vi "获取测试项目和点数.vi"(10 "Item&Count1":string[][](array[string])=[["DCR", "1"], ["DCV", "2"], ["ACV1", "4"], ["ACV2", "4"], ["DCI", "6"], ["ACI", "3"]], 11 "Item":refnum<vi>[](array[refnum])) -> (1 "测量项目":string[](array[string]), 3 "测量点数":i32[](array[numeric]))   [LabVIEW 2020]
panel:
  out "Item&Count2":string[][](array[string])
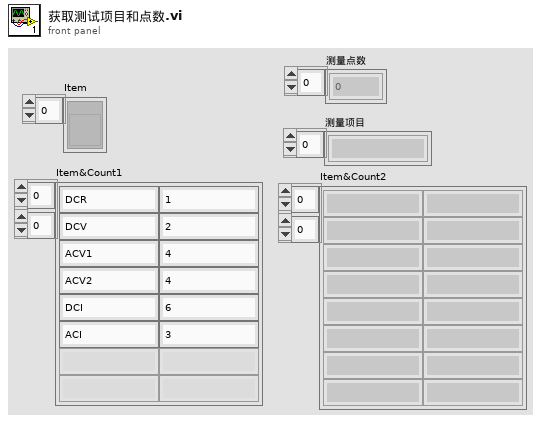
[diagram p1: front panel]
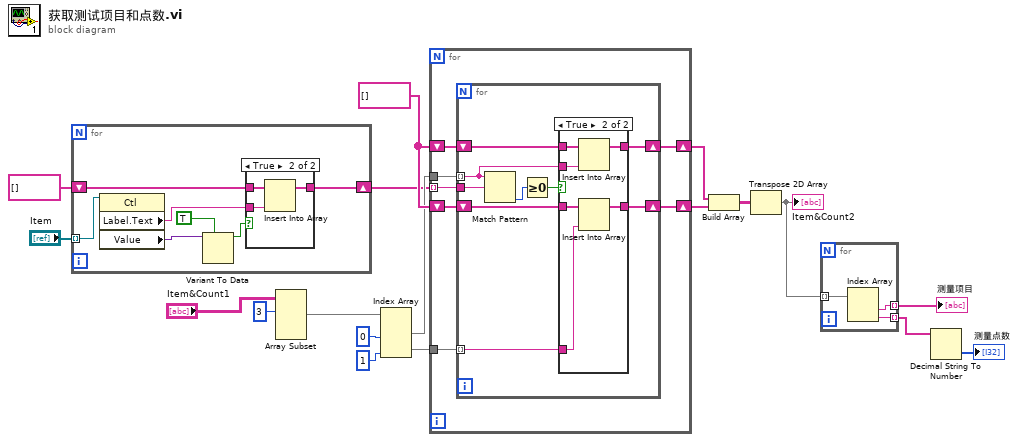
[diagram p0: block diagram]
diagram:
  w15 = string[] [] ("数组")
  n1 = for {
    shift-right: [w20] -> w11
    shift-left: string[] [] ("数组") -> [w21]
    tunnel: "Item" -> [w19] mode=indexing
    n2 = property class="Ctl"(reference=w19) -> ("Label.Text"=w22:string, "Value"=w25:variant)  [unwired: 1 in, 2 out]
    n3 = Variant To Data(type=TRUE, Variant=w25) -> (data=w23:bool)  [unwired: 1 in, 1 out]
    n4 = case shown="True" w23 {
      tunnel: w22 -> [_ w28]
      tunnel: w21 -> [w26 w29]
      tunnel: [w26 w27] -> w20
      frame False {
      }
      frame True {
        n5 = Insert Into Array(array=w29, new element=w28) -> (w27:string[])  [unwired: 1 in]
      }
    }
  }
  n6 = Array Subset(array="Item&Count1", index (row)=3 ("索引")) -> (w5:string[][])  [unwired: 3 in]
  n7 = Index Array(array=w5, index (col) #1=0 ("禁用的索引 (列)"), index (col) #2=1 ("索引 (列)")) -> (element #1=w12:string[], element #2=w14:string[])  [unwired: 2 in]
  n8 = for {
    tunnel: w11 -> [w36] mode=indexing
    tunnel: w12 -> [w35]
    shift-right: [w34] -> w16
    shift-left: w15 -> [w33]
    shift-right: [w31] -> w17
    shift-left: w15 -> [w32]
    tunnel: w14 -> [w30]
    n9 = for {
      tunnel: w36 -> [w45]
      tunnel: w35 -> [w41] mode=indexing
      shift-right: [w40] -> w34
      shift-left: w33 -> [w42]
      shift-right: [w38] -> w31
      shift-left: w32 -> [w39]
      tunnel: w30 -> [w37] mode=indexing
      n10 = Match Pattern(string=w41, regular expression=w45) -> (offset past match=w44:i32)  [unwired: 1 in, 3 out]
      n11 = Greater Or Equal To 0?(x=w44) -> (x >= 0?=w43:bool)
      n12 = case shown="True" w43 {
        tunnel: w42 -> [w47 w53]
        tunnel: w41 -> [_ w52]
        tunnel: [w47 w51] -> w40
        tunnel: w39 -> [w46 w50]
        tunnel: [w46 w49] -> w38
        tunnel: w37 -> [_ w48]
        frame False {
        }
        frame True {
          n13 = Insert Into Array(array=w53, new element=w52) -> (w51:string[])  [unwired: 1 in]
          n14 = Insert Into Array(array=w50, new element=w48) -> (w49:string[])  [unwired: 1 in]
        }
      }
    }
  }
  n15 = Build Array(w16, w17) -> (w18:string[][])
  n16 = Transpose 2D Array(2D array=w18) -> (transposed array=w4:string[][])
  "Item&Count2" <- w4
  n17 = for {
    tunnel: w4 -> [w56] mode=indexing
    tunnel: [w55] -> w1 mode=indexing
    tunnel: [w54] -> w3 mode=indexing
    n18 = Index Array(array=w56) -> (element #1=w55:string, element #2=w54:string)  [unwired: 2 in]
  }
  "测量项目" <- w1
  n19 = Decimal String To Number(string=w3) -> (number=→"测量点数":i32[])  [unwired: 2 in, 1 out]
